vi "Get DB-Type.vi"(6 "wait for reply (T)":bool=TRUE, 8 "error in (no error)":errorcluster, 11 "Module ID":i32=-1) -> (0 "error out":errorcluster, 3 "DB-Type":string)   [LabVIEW 2020, in "hse-db.lvlib" / "DB_CONNECTOR.lvlib"]
doc: "Returns the type of the database in <b>DB-Type</b>\n____\nHAMPEL SOFTWARE ENGINEERING v1.4.0 (2023-12-19 09:52)"
uses:
  DB_CONNECTOR.lvlib
  Get DB-Type Argument--cluster.ctl
  Get DB-Type (Reply Payload)--cluster.ctl
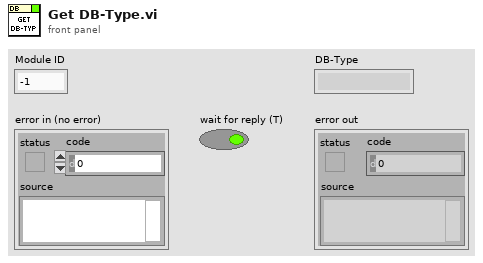
[diagram p1: front panel]
types:
  T1 = typedef "hse-db.lvlib/DB_CONNECTOR.lvlib/Get DB-Type Argument--cluster.ctl" = cluster{"Module ID":i32, "Wait Notifier":refnum<notifier>, "wait for reply":bool}
  T2 = typedef "hse-db.lvlib/DB_CONNECTOR.lvlib/Request Events--cluster.ctl" = cluster{"Stop Module":refnum<user-event>, "Show Panel":refnum<user-event>, "Hide Panel":refnum<user-event>, "Show Diagram":refnum<user-event>, "Get Module Execution Status":refnum<user-event>, "Configure":refnum<user-event>, "Connect":refnum<user-event>, "Close Connection":refnum<user-event>, "Start Transaction":refnum<user-event>, "Fast Query":refnum<user-event>, "Get DB-Type":refnum<user-event>, "Query":refnum<user-event>, "Commit Transaction":refnum<user-event>, "Set Module Timeout":refnum<user-event>, "Rollback Transaction":refnum<user-event>}
  T3 = typedef "hse-db.lvlib/DB_CONNECTOR.lvlib/Get DB-Type (Reply Payload)--cluster.ctl" = cluster{"DB-Type":string, "error":errorcluster, "Module ID":i32}
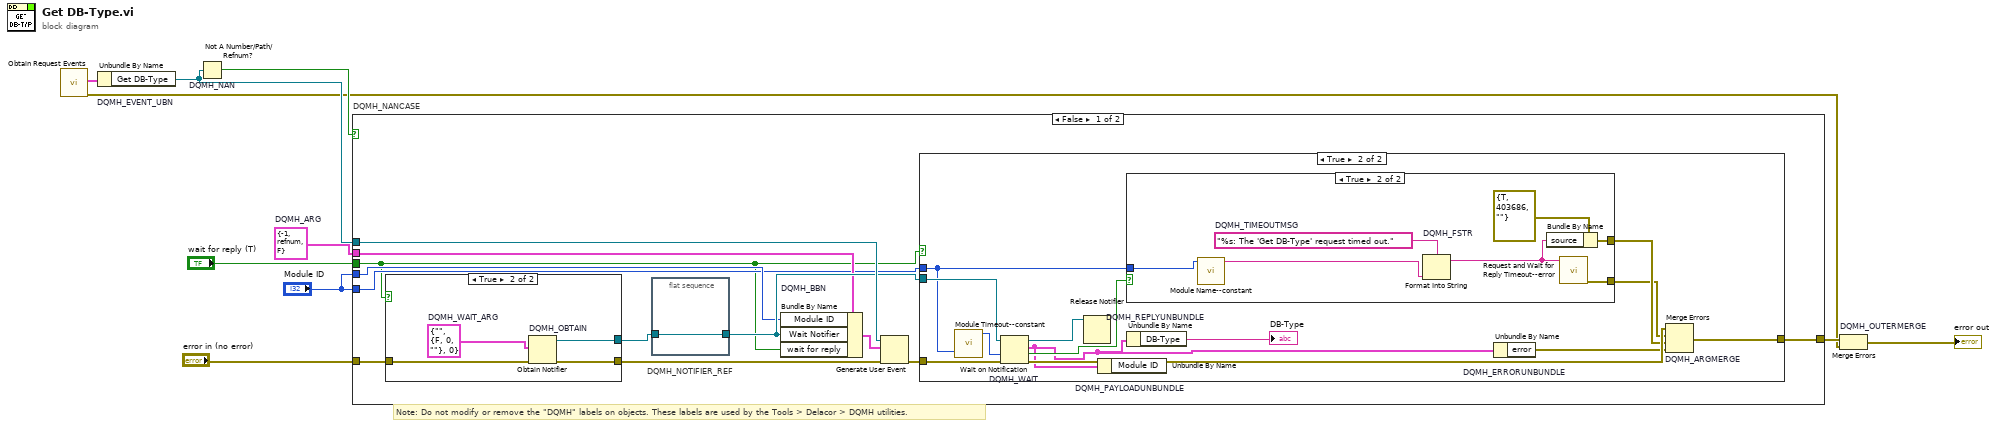
[diagram p0: block diagram]
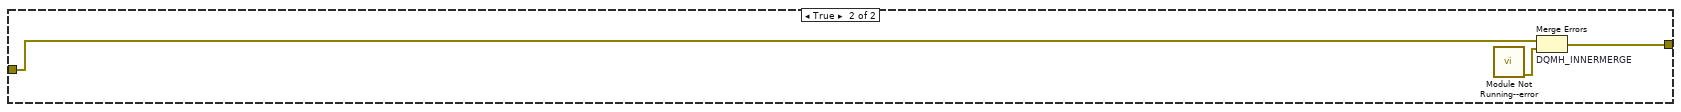
[diagram p5: hidden frame]
diagram:
  w5 = T1 {"Module ID"=-1, "Wait Notifier"=refnum, "wait for reply"=FALSE}  # DQMH_ARG
  # "Note: Do not modify or remove the \"DQMH\" labels on objects. These labels are used by the Tools > Delacor > DQMH utilities."
  n1 = call "Obtain Request Events.vi"() -> ("error out"=w2:errorcluster, "DB_CONNECTOR Request Events"=w1:T2)  [unwired: 10 in]
  n2 = Unbundle By Name "DQMH_EVENT_UBN"(w1) -> ("Get DB-Type"=w8:refnum<user-event>)
  n3 = Not A Number/Path/Refnum? "DQMH_NAN"(number/path/refnum=w8) -> (NaN/Path/Refnum?=w7:bool)
  n4 = case "DQMH_NANCASE" shown="False" w7 {
    tunnel: "error in (no error)" -> [w22 w52]
    tunnel: w8 -> [w20 _]
    tunnel: [w18 w51] -> w6
    tunnel: w5 -> [w14 _]
    tunnel: "Module ID" -> [w13 _]
    tunnel: "Module ID" -> [w12 _]
    tunnel: "wait for reply (T)" -> [w11 _]
    frame False {
      n5 = case shown="True" w11 {
        tunnel: w22 -> [w45 w49]
        tunnel: [w45 w48] -> w19
        tunnel: [_ w46] -> w16
        frame False {
        }
        frame True {
          w47 = T3 {"DB-Type"="", "error"={"status"=FALSE, "code"=0, "source"=""}, "Module ID"=0}  # DQMH_WAIT_ARG
          n6 = Obtain Notifier "DQMH_OBTAIN"(notification data type=w47, error in (no error)=w49) -> (notifier out=w46:refnum<notifier>, error out=w48:errorcluster)  [unwired: 2 in, 1 out]
        }
      }
      n7 = flat-sequence "DQMH_NOTIFIER_REF" {
        tunnel: w16 -> [w23]
        tunnel: [w23] -> w15
        frame #0 {
        }
      }
      n8 = Bundle By Name "DQMH_BBN"(cluster=w14, "Module ID"=w13, "Wait Notifier"=w15, "wait for reply"=w11) -> (w17:T1)
      n9 = Generate User Event(user event=w20, event data cluster=w17, error in=w19) -> (error out=w21:errorcluster)  [unwired: 1 in, 1 out]
      n10 = case shown="True" w11 {
        tunnel: w21 -> [w24 w37]
        tunnel: w15 -> [_ w35]
        tunnel: [w24 w32] -> w18
        tunnel: w12 -> [_ w25]
        frame False {
        }
        frame True {
          n11 = call "Module Timeout--constant.vi"("Module ID"=w25) -> ("Module Timeout"=w30:i32)  [unwired: 10 in]
          n12 = Wait on Notification "DQMH_WAIT"(notifier=w35, timeout in ms (-1)=w30, error in (no error)=w37) -> (notifier out=w34:refnum<notifier>, notification=w29:T3, timed out?=w33:bool, error out=w36:errorcluster)  [unwired: 1 in]
          n13 = Release Notifier(notifier=w34) -> ()  [unwired: 2 in, 3 out]
          n14 = Unbundle By Name "DQMH_PAYLOADUNBUNDLE"(w29) -> ()  [unwired: 1 out]
          n15 = case shown="True" w33 {
            tunnel: w25 -> [_ w42]
            tunnel: [_ w39] -> w27
            tunnel: [_ w38] -> w26
            frame False {
            }
            frame True {
              w44 = "%s: The 'Get DB-Type' request timed out."  # DQMH_TIMEOUTMSG
              n16 = call "Module Name--constant.vi"("Module ID"=w42) -> ("Module Name"=w43:string)  [unwired: 10 in]
              n17 = Format Into String "DQMH_FSTR"(format string=w44, w43) -> (resulting string=w40:string)  [unwired: 2 in, 1 out]
              n18 = Bundle By Name(cluster=errorcluster {"status"=TRUE, "code"=403686, "source"=""} ("error in (no error)"), "source"=w40) -> (w39:errorcluster)
              n19 = call "Request and Wait for Reply Timeout--error.vi"("Error Message"=w40) -> ("error out"=w38:errorcluster)  [unwired: 10 in]
            }
          }
          n20 = Unbundle By Name "DQMH_REPLYUNBUNDLE"(w29) -> ("DB-Type"=→"DB-Type":string)
          n21 = Unbundle By Name "DQMH_ERRORUNBUNDLE"(w29) -> ("error"=w31:errorcluster)
          n22 = Merge Errors "DQMH_ARGMERGE"(w36, w26, w27, w31) -> (w32:errorcluster)
        }
      }
    }
    frame True {
      n23 = call "Module Not Running--error.vi"() -> ("error out"=w50:errorcluster)  [unwired: 11 in]
      n24 = Merge Errors "DQMH_INNERMERGE"(w52, w50) -> (w51:errorcluster)
    }
  }
  n25 = Merge Errors "DQMH_OUTERMERGE"(w6, w2) -> (→"error out":errorcluster)
